vi "manage execution errors.vi"(8 "error in (no error)":errorcluster, 11 "Channel in":refnum<class "Channel.lvclass">) -> (0 "error out":errorcluster, 3 "Channel out":refnum<class "Channel.lvclass">)   [LabVIEW 2018, in "Channel.lvclass"]
uses:
  Channel.lvclass
  Channel.lvclass/Channel.ctl
  Error log/Error log.lvclass
  Simulated_CCD_Camera/Simulated Camera.lvclass
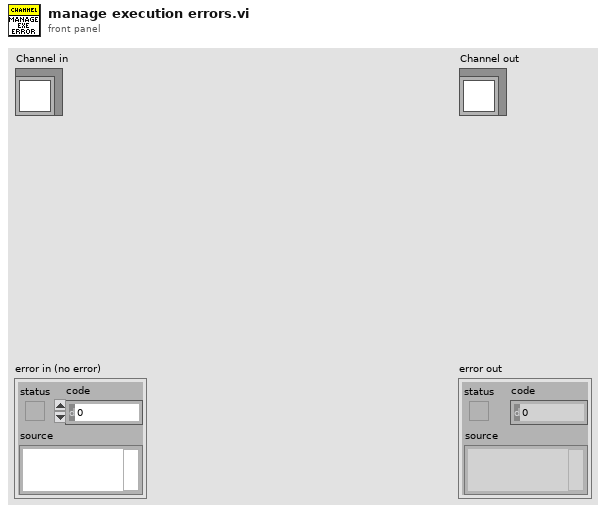
[diagram p1: front panel]
types:
  T1 = cluster{"CYCLES_DONE":u16, "LAST_IMAGE_NAME":string, "USED_DISK_SPACE":u16, "FRAMES_DONE":u16, "CCD_STATUS":string, "CURRENT_TEMPERATURE":i16, "TEMPERATURE_STATUS":string, "FRAME_EXPOSURE_TIME":sgl, "ERROR":bool, "SERIAL_NUMBER":u16, "ACQUIRING":bool, "IMAGE_INDEX":u32, "SEQS_DONE":u16}
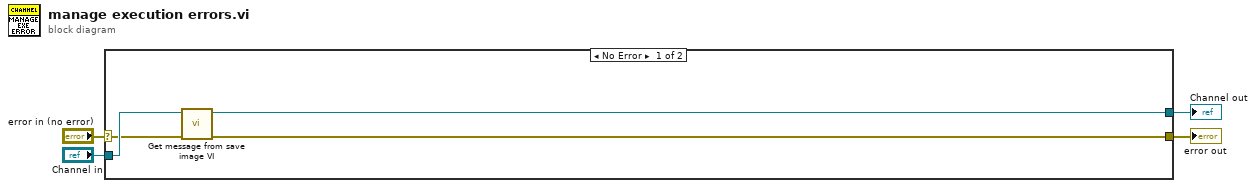
[diagram p0: block diagram]
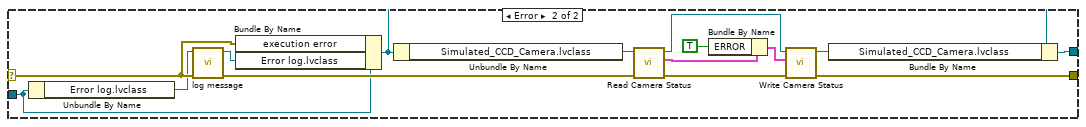
[diagram p2: hidden frame]
diagram:
  n1 = case shown="No Error" "error in (no error)" {
    selector: "error in (no error)" -> [w5 w13]
    tunnel: [w6 w14] -> w4
    tunnel: [w7 w10] -> w3
    tunnel: "Channel in" -> [w8 w11]
    frame No Error {
      n2 = call "Get message from save image VI.vi"("error in (no error)"=w5, "Channel in"=w8) -> ("error out"=w6:errorcluster, "Channel out"=w7:refnum<class "Channel.lvclass">)  [unwired: 8 in]
    }
    frame Error {
      n3 = Unbundle By Name(w11) -> ("Error log.lvclass"=w12:refnum<class "Error log.lvclass">)
      n4 = call-dynamic "log message.vi"("error in (no error)"=w13, "Error log in"=w12) -> ("error out"=w20:errorcluster, "Error log out"=w23:refnum<class "Error log.lvclass">)  [unwired: 8 in]
      n5 = Bundle By Name(cluster=w11, "execution error"=w13, "Error log.lvclass"=w23) -> (w15:refnum<class "Channel.lvclass">)
      n6 = Unbundle By Name(w15) -> ("Simulated_CCD_Camera.lvclass"=w9:refnum<class "Simulated Camera.lvclass">)
      n7 = call "Read Camera Status.vi"("error in (no error)"=w20, "CCDCamera in"=w9) -> ("error out"=w19:errorcluster, "Camera Status"=w17:T1, "CCDCamera out"=w22:refnum<class "Simulated Camera.lvclass">)  [unwired: 7 in]
      n8 = Bundle By Name(cluster=w17, "ERROR"=TRUE) -> (w18:T1)
      n9 = call "Write Camera Status.vi"("error in (no error)"=w19, "Camera Status"=w18, "CCDCamera in"=w22) -> ("error out"=w14:errorcluster, "CCDCamera out"=w21:refnum<class "Simulated Camera.lvclass">)  [unwired: 7 in]
      n10 = Bundle By Name(cluster=w15, "Simulated_CCD_Camera.lvclass"=w21) -> (w10:refnum<class "Channel.lvclass">)
    }
  }
  "error out" <- w4
  "Channel out" <- w3
